vi "Asserts.vi"(0 "VI Reference In":refnum<vi>, 1 "Label (VI Title)":string="Default", 11 "error in (no error)":errorcluster) -> (4 "VI Reference Out":refnum<vi>, 15 "error out":errorcluster)   [LabVIEW 2016, in "Drona Test.lvlib"]
uses:
  Drona Test.lvlib
  main/apis/Stimulus/KeyBoardSimulation/ValueSignalLatchBooleanString.vi
  main/apis/Assert/AssertControlValue/Greater.vi
  <vilib>/addons/_JKI Toolkits/Caraya/classes/Assert/Assert Error.vi
  main/apis/Assert/AssertControlValue/AlmostEqual.vi
  <vilib>/addons/_JKI Toolkits/Caraya/classes/Assert/Assert Not Error.vi
  <vilib>/addons/_JKI Toolkits/Caraya/classes/Test/Test.lvclass
  main/Drona.lvlib
  <vilib>/addons/_JKI Toolkits/Caraya/classes/Assert/Assert.lvclass
  main/apis/Stimulus/KeyBoardSimulation/KeyboardSimulation.lvlib
  main/apis/Assert/AssertControlValue/AssertControlValue.lvlib
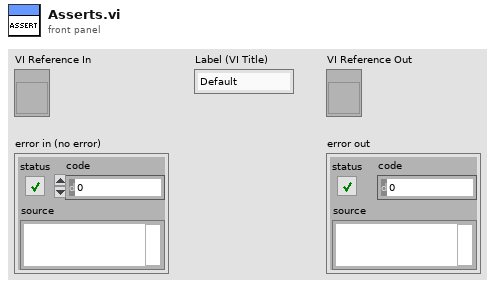
[diagram p1: front panel]
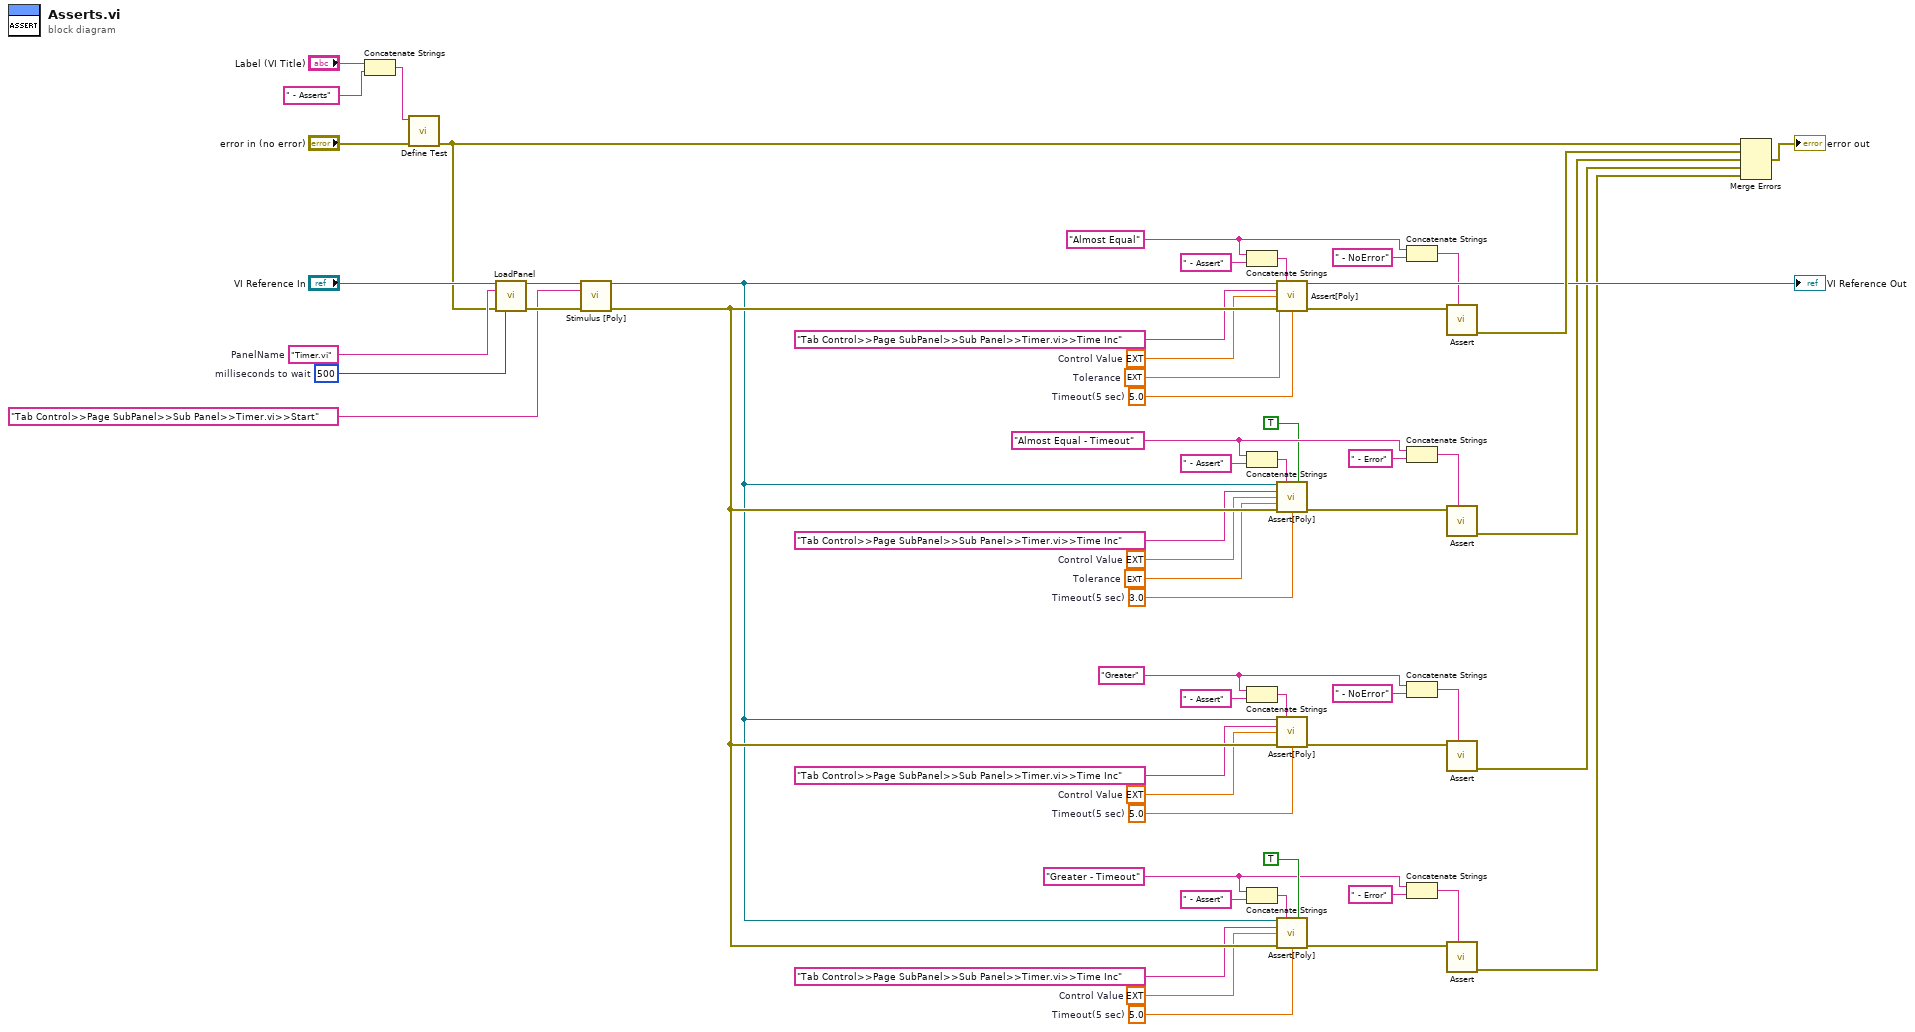
[diagram p0: block diagram]
diagram:
  w9 = 5.0  # Timeout(5 sec)
  w8 = ext 3.0  # Control Value
  w7 = "Greater" ("string")
  w10 = ext 0.5  # Tolerance
  w11 = ext 0.5  # Tolerance
  w21 = 3.0  # Timeout(5 sec)
  w20 = ext 5.0  # Control Value
  w19 = "Almost Equal - Timeout" ("string")
  w22 = 5.0  # Timeout(5 sec)
  w23 = ext 5.0  # Control Value
  w24 = "Almost Equal" ("string")
  w31 = 5.0  # Timeout(5 sec)
  w32 = ext 15.0  # Control Value
  w33 = "Greater - Timeout" ("string")
  w48 = u32 500  # milliseconds to wait
  w52 = "Timer.vi"  # PanelName
  n1 = Concatenate Strings("Label (VI Title)", " - Asserts" ("Label (VI Title)")) -> (w54:string)
  n2 = call <vilib>:"Define Test.vi"("error in (no error)"="error in (no error)", "Label (VI Title)"=w54) -> ("error out"=w45:errorcluster)  [unwired: 9 in]
  n3 = call "LoadPanel.vi"("VI in"="VI Reference In", "Panel Name"=w52, "error in (no error)"=w45, "milliseconds to wait"=w48) -> ("VI out"=w51:refnum<vi>, "error out"=w49:errorcluster)  [unwired: 10 in]
  n4 = call-poly "Stimulus [Poly].vi"("VI Reference In"=w51, "Control Path"="Tab Control>>Page SubPanel>>Sub Panel>>Timer.vi>>Start", "error in"=w49) -> ("VI Reference Out"=w43:refnum<vi>, "error out"=w44:errorcluster)  [unwired: 11 in]
  n5 = Concatenate Strings(w24, " - Assert" ("string")) -> (w26:string)
  n6 = Concatenate Strings(w19, " - Assert" ("string")) -> (w17:string)
  n7 = Concatenate Strings(w7, " - Assert" ("string")) -> (w5:string)
  n8 = Concatenate Strings(w33, " - Assert" ("string")) -> (w35:string)
  n9 = call-poly "Assert[Poly].vi"("VI Reference In"=w43, "Label"=w26, "Control Path"="Tab Control>>Page SubPanel>>Sub Panel>>Timer.vi>>Time Inc", "Control Value"=w23, "Tolerance"=w11, "Error In"=w44, "Timeout(5 sec)"=w22) -> ("VI Reference Out"=→"VI Reference Out":refnum<vi>, "Error Out"=w27:errorcluster)  [unwired: 7 in]
  n10 = call-poly "Assert[Poly].vi"("VI Reference In"=w43, "Label"=w17, "Assert Only? (F)"=TRUE, "Control Path"="Tab Control>>Page SubPanel>>Sub Panel>>Timer.vi>>Time Inc", "Control Value"=w20, "Tolerance"=w10, "Error In"=w44, "Timeout(5 sec)"=w21) -> ("Error Out"=w16:errorcluster)  [unwired: 6 in, 1 out]
  n11 = call-poly "Assert[Poly].vi"("VI Reference In"=w43, "Label"=w5, "Control Path"="Tab Control>>Page SubPanel>>Sub Panel>>Timer.vi>>Time Inc", "Control Value"=w8, "Error In"=w44, "Timeout(5 sec)"=w9) -> ("Error Out"=w4:errorcluster)  [unwired: 8 in, 1 out]
  n12 = call-poly "Assert[Poly].vi"("VI Reference In"=w43, "Label"=w35, "Assert Only? (F)"=TRUE, "Control Path"="Tab Control>>Page SubPanel>>Sub Panel>>Timer.vi>>Time Inc", "Control Value"=w32, "Error In"=w44, "Timeout(5 sec)"=w31) -> ("Error Out"=w36:errorcluster)  [unwired: 7 in, 1 out]
  n13 = Concatenate Strings(w24, " - NoError" ("string")) -> (w25:string)
  n14 = Concatenate Strings(w19, " - Error" ("string")) -> (w18:string)
  n15 = Concatenate Strings(w7, " - NoError" ("string")) -> (w6:string)
  n16 = Concatenate Strings(w33, " - Error" ("string")) -> (w34:string)
  n17 = call-poly <vilib>:"Assert.vi"("Label"=w25, "Not Error?"=w27) -> ("error out"=w59:errorcluster)  [unwired: 9 in]
  n18 = call-poly <vilib>:"Assert.vi"("Label"=w18, "Error?"=w16) -> ("error out"=w46:errorcluster)  [unwired: 9 in]
  n19 = call-poly <vilib>:"Assert.vi"("Label"=w6, "Not Error?"=w4) -> ("error out"=w42:errorcluster)  [unwired: 9 in]
  n20 = call-poly <vilib>:"Assert.vi"("Label"=w34, "Error?"=w36) -> ("error out"=w41:errorcluster)  [unwired: 9 in]
  n21 = Merge Errors(w45, w59, w46, w42, w41) -> (→"error out":errorcluster)
